vi "k5_Create.vi"(6 "deviceType":T1, 8 "error in (no error)":errorcluster, 9 "dim":i32, 10 "index":i32, 11 "reference in":refnum<class "k5.lvclass">) -> (0 "error out":errorcluster, 3 "reference out":refnum<class "k5.lvclass">)   [LabVIEW 2014, in "k5.lvclass"]
doc: "Constructor."
uses:
  k5.lvclass
  SYS/Devices Controller_llb/deviceType.ctl
  <vilib>/addons/_AddQ/G#Object/utils/G#Object_CreateMethod.ctl
  <vilib>/addons/_AddQ/G#Object/G#Object.lvclass
  SYS/Devices Controller_llb/Devices Controller.lvclass
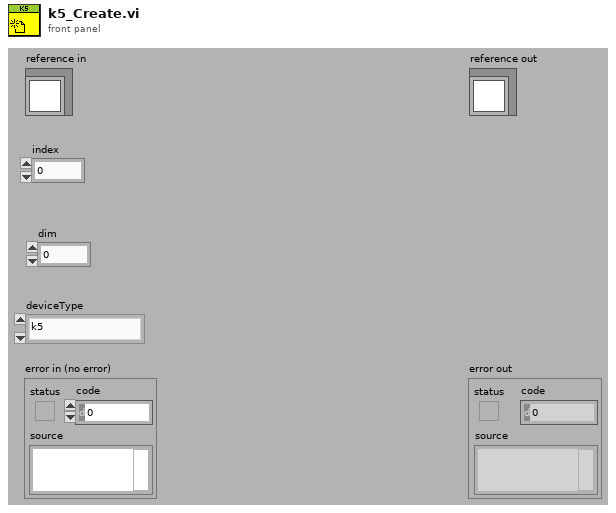
[diagram p1: front panel]
types:
  T1 = typedef "Devices Controller.lvclass/deviceType.ctl" = enum16{"k5", "k4b2", "fitmate", "cpet", "rmr", "bodyBoxPft", "bp", "pp"}
  T2 = typedef "G#Object.lvclass/G#Object_CreateMethod.ctl" = enum16{"Create", "Create or look up existing", "Look up existing"}
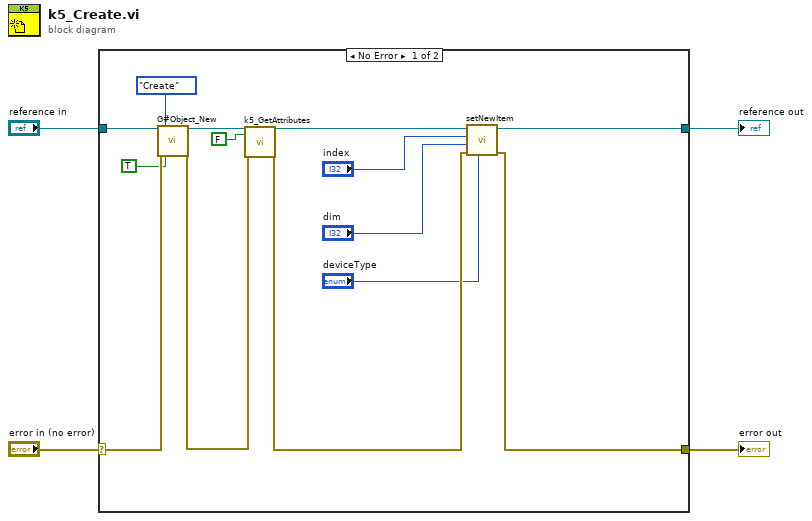
[diagram p0: block diagram]
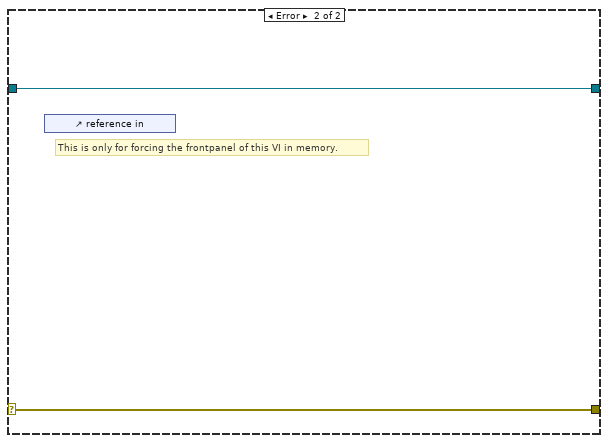
[diagram p2: hidden frame]
diagram:
  n1 = case shown="No Error" "error in (no error)" {
    selector: "error in (no error)" -> [w17 w20]
    tunnel: [w10 w20] -> w3
    tunnel: [w8 w19] -> w1
    tunnel: "reference in" -> [w18 w19]
    frame No Error {
      n2 = call <vilib>:"G#Object_New.vi"("reference in"=w18, "error in (no error)"=w17, "create method"=G#Object_CreateMethod."Create", "user counter (T)?"=TRUE ("User Counter")) -> ("reference out"=w15:refnum<class "k5.lvclass">, "error out"=w14:errorcluster)  [unwired: 13 in, 1 out]
      n3 = call "k5_GetAttributes.vi"("reference in"=w15, "return data? (T)"=FALSE ("return data"), "error in (no error)"=w14) -> ("reference out"=w9:refnum<class "k5.lvclass">, "error out"=w11:errorcluster)  [unwired: 13 in, 2 out]
      n4 = call "setNewItem.vi"("deviceType"="deviceType", "error in (no error)"=w11, "dim"="dim", "index"="index", "reference in"=w9) -> ("error out"=w10:errorcluster, "reference out"=w8:refnum<class "k5.lvclass">)  [unwired: 5 in]
    }
    frame Error {
      # "This is only for forcing the frontpanel of this VI in memory."
      n5 = control-ref of="reference in"() -> ()  [unwired: 1 out]
    }
  }
  "error out" <- w3
  "reference out" <- w1
